vi "TemperatureStub.vi"(6 "TemperatureIn":dbl[](array[numeric]), 8 "error in":errorcluster, 9 "Length":i32=250, 11 "ON":bool) -> (0 "error out":errorcluster, 1 "TemperatureOut":dbl[](array[numeric]))   [LabVIEW 2012]
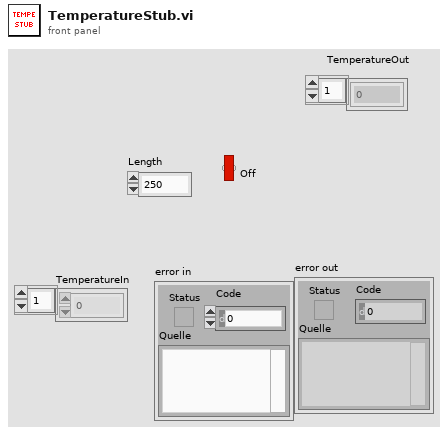
[diagram p1: front panel]
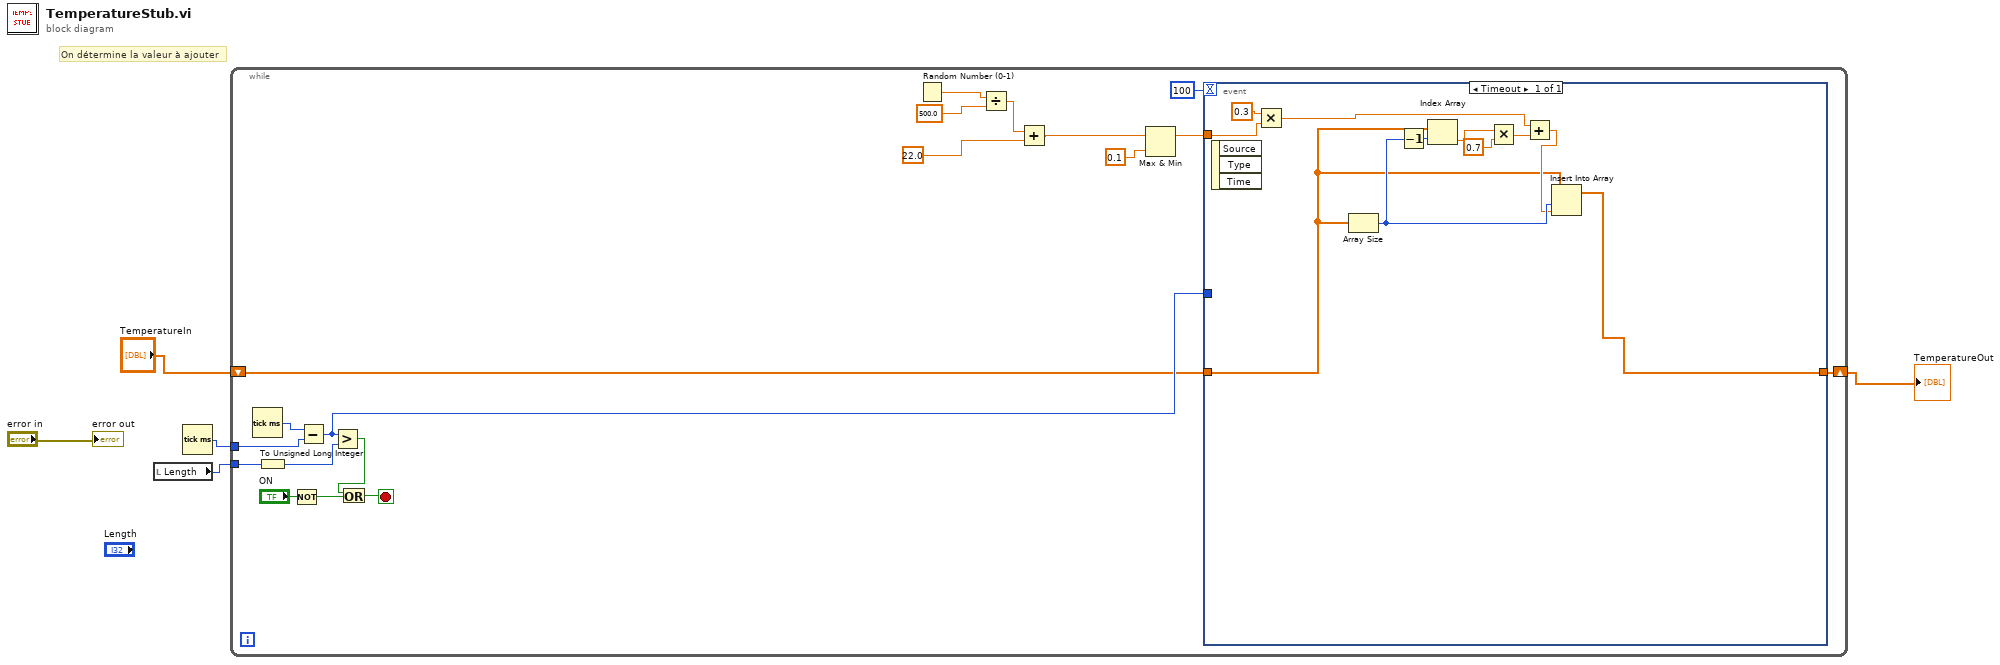
[diagram p0: block diagram]
diagram:
  # "On détermine la valeur à ajouter"
  n1 = local read "Length"() -> (w4:i32)
  n2 = Tick Count (ms)() -> (millisecond timer value=w5:u32)
  n3 = while {
    tunnel: w5 -> [w20]
    tunnel: w4 -> [w16]
    shift-right: [w6] -> w1
    shift-left: "TemperatureIn" -> [w7]
    stop <- w22 stop-if-true
    n4 = Tick Count (ms)() -> (millisecond timer value=w21:u32)
    n5 = To Unsigned Long Integer(number=w16) -> (unsigned 32bit integer=w15:u32)
    n6 = Not(x="ON") -> (.not. x?=w23:bool)
    n7 = Subtract(x=w21, y=w20) -> (x-y=w17:u32)
    n8 = Greater?(x=w17, y=w15) -> (0:w19:bool)
    n9 = Or(x=w19, y=w23) -> (x .or. y?=w22:bool)
    n10 = Random Number (0-1)() -> (number: 0 to 1=w13:dbl)
    n11 = Divide(x=w13, y=500.0) -> (x/y=w12:dbl)
    n12 = Add(x=w12, y=22.0) -> (x+y=w9:dbl)
    n13 = Max & Min(x=w9, y=0.1) -> (max(x,y)=w11:dbl)  [unwired: 1 out]
    n14 = event shown="[0] Timeout" {
      selector: _ -> [_]
      dyn-events: _ -> [_]
      timeout: 100 -> [_]
      tunnel: w17 -> [_]
      tunnel: w11 -> [w31]
      tunnel: w7 -> [w26]
      tunnel: [w25] -> w6
      event Timeout {
        n15 = event-data() -> ()  [unwired: 1 in, 3 out]
        n16 = Multiply(x=0.3, y=w31) -> (x*y=w29:dbl)
        n17 = Array Size(array=w26) -> (size(s)=w34:i32)
        n18 = Decrement(x=w34) -> (x-1=w35:i32)
        n19 = Index Array(array=w26, index=w35) -> (element=w28:dbl)
        n20 = Multiply(x=w28, y=0.7) -> (x*y=w30:dbl)
        n21 = Add(x=w29, y=w30) -> (x+y=w27:dbl)
        n22 = Insert Into Array(array=w26, index=w34, new element=w27) -> (w25:dbl[])
      }
    }
  }
  "TemperatureOut" <- w1
  "error out" <- "error in"
